vi "Labview_Database_try - backup.vi"() -> ()   [LabVIEW 2012]
uses:
  <vilib>/addons/database/Connection.llb/DB Tools Open Connec (Path).vi
  <vilib>/addons/database/NI_Database_API.lvlib
panel:
  out "Pressure-Time Plot":cluster{dbl[], dbl[]}(graph)
  in  "Start time":timestamp
  in  "End time":timestamp
  out "Temperature-Time Plot":cluster{dbl[], dbl[]}(graph)
  out "data":string[][](table)
  out "error out":errorcluster
  in  "Table chosen":string
  in  "stop":bool
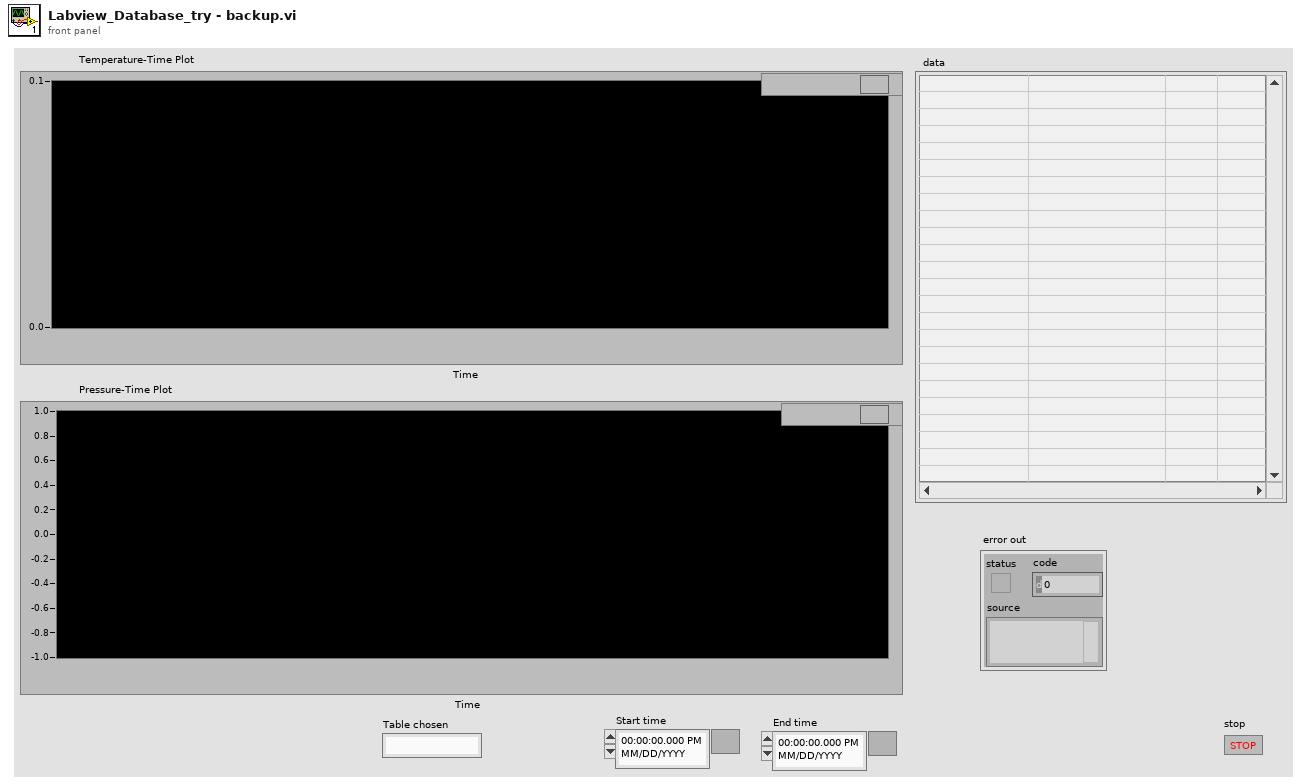
[diagram p1: front panel]
types:
  T1 = typedef "NI_Database_API.lvlib/Conn ObjectReference.ctl" = refnum<k1>
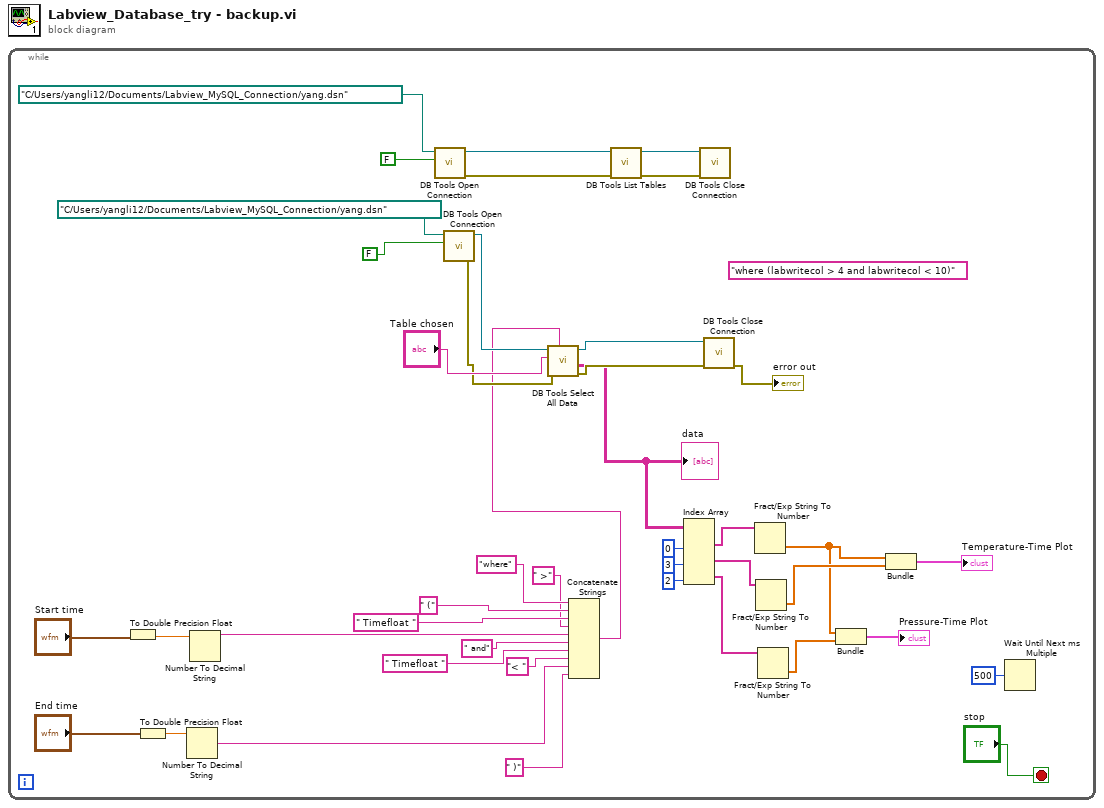
[diagram p0: block diagram]
diagram:
  n1 = while {
    stop <- "stop" stop-if-true
    (unwired) "where (labwritecol > 4 and labwritecol < 10)" ("condition")
    n2 = To Double Precision Float(number="Start time") -> (double precision float=w14:dbl)
    n3 = To Double Precision Float(number="End time") -> (double precision float=w9:dbl)
    n4 = Number To Decimal String(number=w9) -> (decimal integer string=w8:string)  [unwired: 1 out]
    n5 = Number To Decimal String(number=w14) -> (decimal integer string=w13:string)  [unwired: 1 out]
    n6 = call-poly <vilib>:"DB Tools Open Connection.vi"("prompt? (F)"=FALSE, "connection information"=path "C:/Users/yangli12/Documents/Labview_MySQL_Connection/yang.dsn") -> ("error out"=w36:errorcluster, "connection reference"=w37:T1)  [unwired: 6 in]
    n7 = call-poly <vilib>:"DB Tools Open Connection.vi"("prompt? (F)"=FALSE, "connection information"=path "C:/Users/yangli12/Documents/Labview_MySQL_Connection/yang.dsn") -> ("error out"=w30:errorcluster, "connection reference"=w32:T1)  [unwired: 6 in]
    n8 = Concatenate Strings("where", " (", " Timefloat " ("string"), " >" ("string"), w13, " and", " Timefloat ", "< " ("string"), w8, " )") -> (w6:string)
    n9 = call <vilib>:"DB Tools Select All Data.vi"("optional clause"=w6, "error in (no error)"=w30, "table"="Table chosen", "connection reference"=w32) -> ("error out"=w29:errorcluster, "data"=w27:string[][], "connection reference out"=w28:T1)  [unwired: 1 in, 1 out]
    "data" <- w27
    n10 = call <vilib>:"DB Tools List Tables.vi"("error in (no error)"=w36, "connection reference"=w37) -> ("error out"=w41:errorcluster, "connection reference out"=w42:T1)  [unwired: 3 in, 1 out]
    n11 = Index Array(array=w27, index (col) #1=0 ("disabled index (col)"), index (col) #2=3 ("index (col)"), index (col) #3=2 ("index (col)")) -> (element #1=w24:string[], element #2=w23:string[], element #3=w5:string[])  [unwired: 3 in]
    n12 = call <vilib>:"DB Tools Close Connection.vi"("error in (no error)"=w41, "connection reference"=w42) -> ()  [unwired: 5 in, 1 out]
    n13 = call <vilib>:"DB Tools Close Connection.vi"("error in (no error)"=w29, "connection reference"=w28) -> ("error out"=→"error out":errorcluster)  [unwired: 5 in]
    n14 = Fract/Exp String To Number(string=w24) -> (number=w4:dbl[])  [unwired: 4 out]
    n15 = Fract/Exp String To Number(string=w23) -> (number=w22:dbl[])  [unwired: 4 out]
    n16 = Fract/Exp String To Number(string=w5) -> (number=w3:dbl[])  [unwired: 4 out]
    n17 = Bundle "Bundle"(w4, w3) -> (→"Pressure-Time Plot":cluster{dbl[], dbl[]})  [unwired: 1 in]
    n18 = Bundle "Bundle"(w4, w22) -> (→"Temperature-Time Plot":cluster{dbl[], dbl[]})  [unwired: 1 in]
    n19 = Wait Until Next ms Multiple(millisecond multiple=u32 500) -> ()  [unwired: 1 out]
  }
